vi "MDI-CSM.vi"(7 "Name (\"\" to Use UUID)":string="Event CSM") -> ()   [LabVIEW 2020]
uses:
  Ctl/View.ctl
  <vilib>/Utility/miscctls.llb/LVPoint32TypeDef.ctl
  Ctl/UpdateInsertableVICtl.ctl
  <vilib>/Utility/miscctls.llb/LVPointTypeDef.ctl
  e5d725f2-e4a0-42ba-b3f6-a9ce6c833174.vi
  4b9b3096-98ee-4c27-a851-eb0343d389bf.vi
  ccb737c0-95ef-485f-9e6a-728d6ff02605.vi
  5110686f-90b8-48a6-8112-abce107b1655.vi
  <userlib>/_NEVSTOP/Communicable State Machine(CSM)/AdvanceAPI/CSM - Revert Arguments-Safe String.vi
  <userlib>/_NEVSTOP/Communicable State Machine(CSM)/_Shared/Trim Single-line Text.vi
  <userlib>/_NEVSTOP/Communicable State Machine(CSM)/AdvanceAPI/CSM - Make String Arguments Safe.vi
  <userlib>/_NEVSTOP/Communicable State Machine(CSM)/AdvanceAPI/CSM - Break Down Multiple States String.vi
  <userlib>/_NEVSTOP/Communicable State Machine(CSM)/AdvanceAPI/CSM - Compact Multiple States.vi
  <userlib>/_NEVSTOP/Communicable State Machine(CSM)/AdvanceAPI/CSM - Keywords.vi
  <vilib>/Utility/cursorutil.llb/Set Cursor (Icon Pict).vi
  <userlib>/_NEVSTOP/Communicable State Machine(CSM)/addons/API-String-Arugments-Support/_Support/Convert API String Arguments to Data(variant).vi
  <userlib>/_NEVSTOP/Communicable State Machine(CSM)/Communicable State Machine.lvlib
panel:
  in  "Tab Control 6":T1
  in  "Tab Control 5":T1
  in  "Tab Control 4":T1
  in  "Tab Control 3":T1
  in  "Tab Control 2":T1
  in  "Tab Control":T1
  out "State History":string
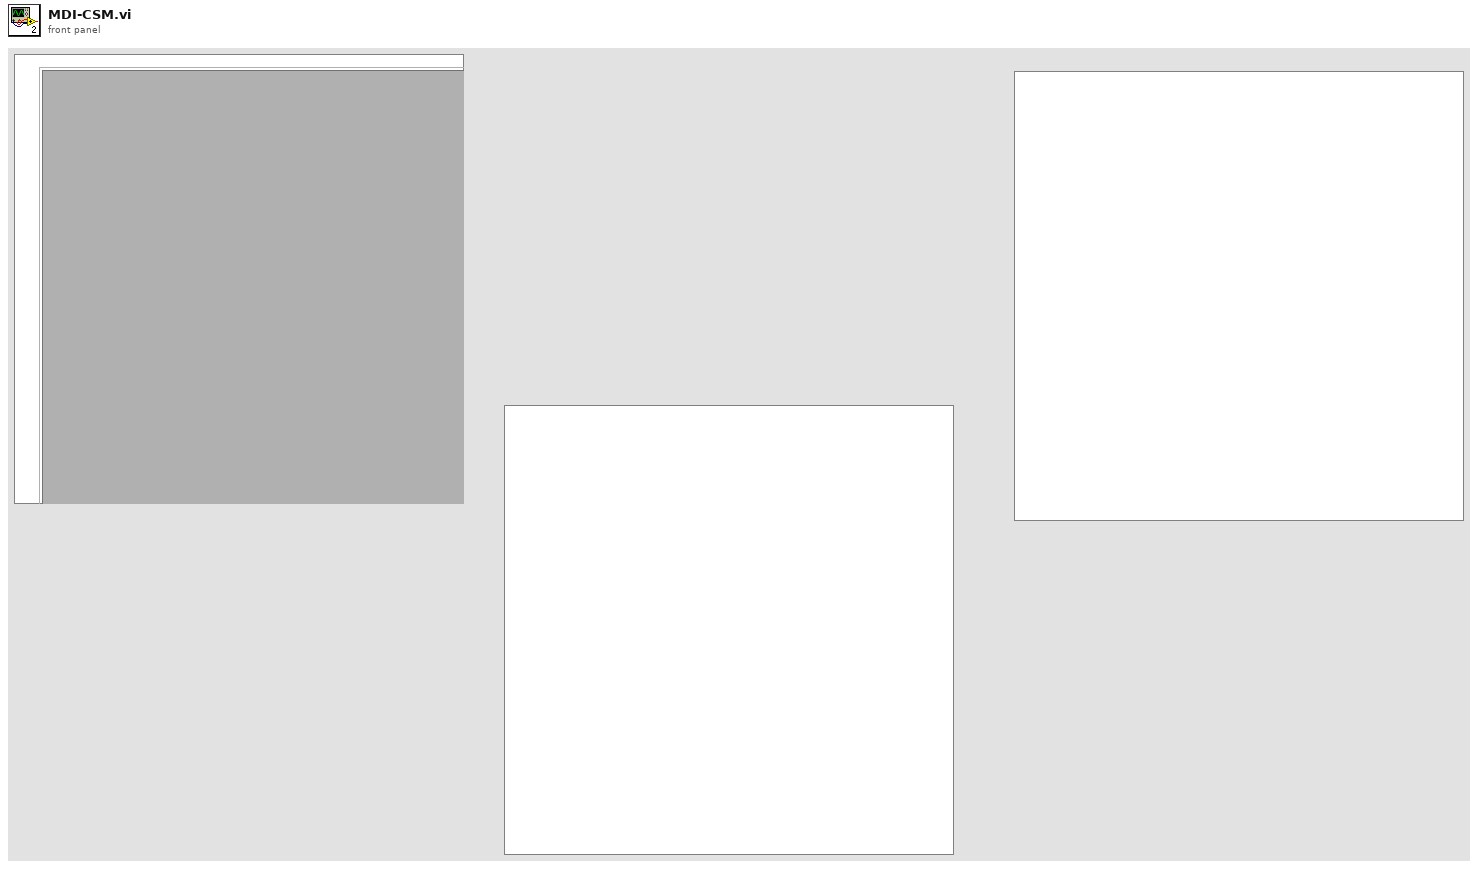
[diagram p1: front panel]
types:
  T1 = typedef "View.ctl" = enum32{"Page 1", "Page 2"}
  T2 = typedef "LVPointTypeDef.ctl" = cluster{"Horizontal":i16, "Vertical":i16}
  T3 = typedef "LVPoint32TypeDef.ctl" = cluster{"Horizontal":i32, "Vertical":i32}
  T4 = typedef "UpdateInsertableVICtl.ctl" = cluster{"Name":string, "VIPath":path}
  T5 = cluster{"Ref":cluster{"TabCtl":refnum<vi>[], "CurrMoveCtl":refnum<vi>, "Pane":refnum<vi>, "SubPanel":refnum<vi>, "Owning VI":refnum<vi>}, "Val":cluster{"TabCtlMove?":bool, "MouseOffset":T3, "UpdateInsertableVI":T4[]}}
  T6 = cluster{"Current VI Reference":refnum<vi>, "Close Panel on Exit?":bool}
  T7 = cluster{"Core":cluster{"Current VI Reference":refnum<vi>, "Close Panel on Exit?":bool}, "1":cluster{"Ref":cluster{"TabCtl":refnum<vi>[], "CurrMoveCtl":refnum<vi>, "Pane":refnum<vi>, "SubPanel":refnum<vi>, "Owning VI":refnum<vi>}, "Val":cluster{"TabCtlMove?":bool, "MouseOffset":T3, "UpdateInsertableVI":T4[]}}}
  T8 = enum32{"Invalid", "Standard", "Closed", "Hidden", "Minimized", "Maximized"}
  T9 = enum32{"invalid app kind", "Development System", "Run Time System", "Student Edition", "Embedded LabVIEW", "Evaluation", "Custom"}
  T10 = typedef "Communicable State Machine.lvlib/_CSM_Response Source Message.ctl" = cluster{"‘State":string, "’Arguments":string, "’Error":errorcluster}
  T11 = typedef "LVPositionTypeDef.ctl" = cluster{"Left":i32, "Top":i32}
  T12 = cluster{"TabCtl":refnum<vi>[], "Pane":refnum<vi>, variant}
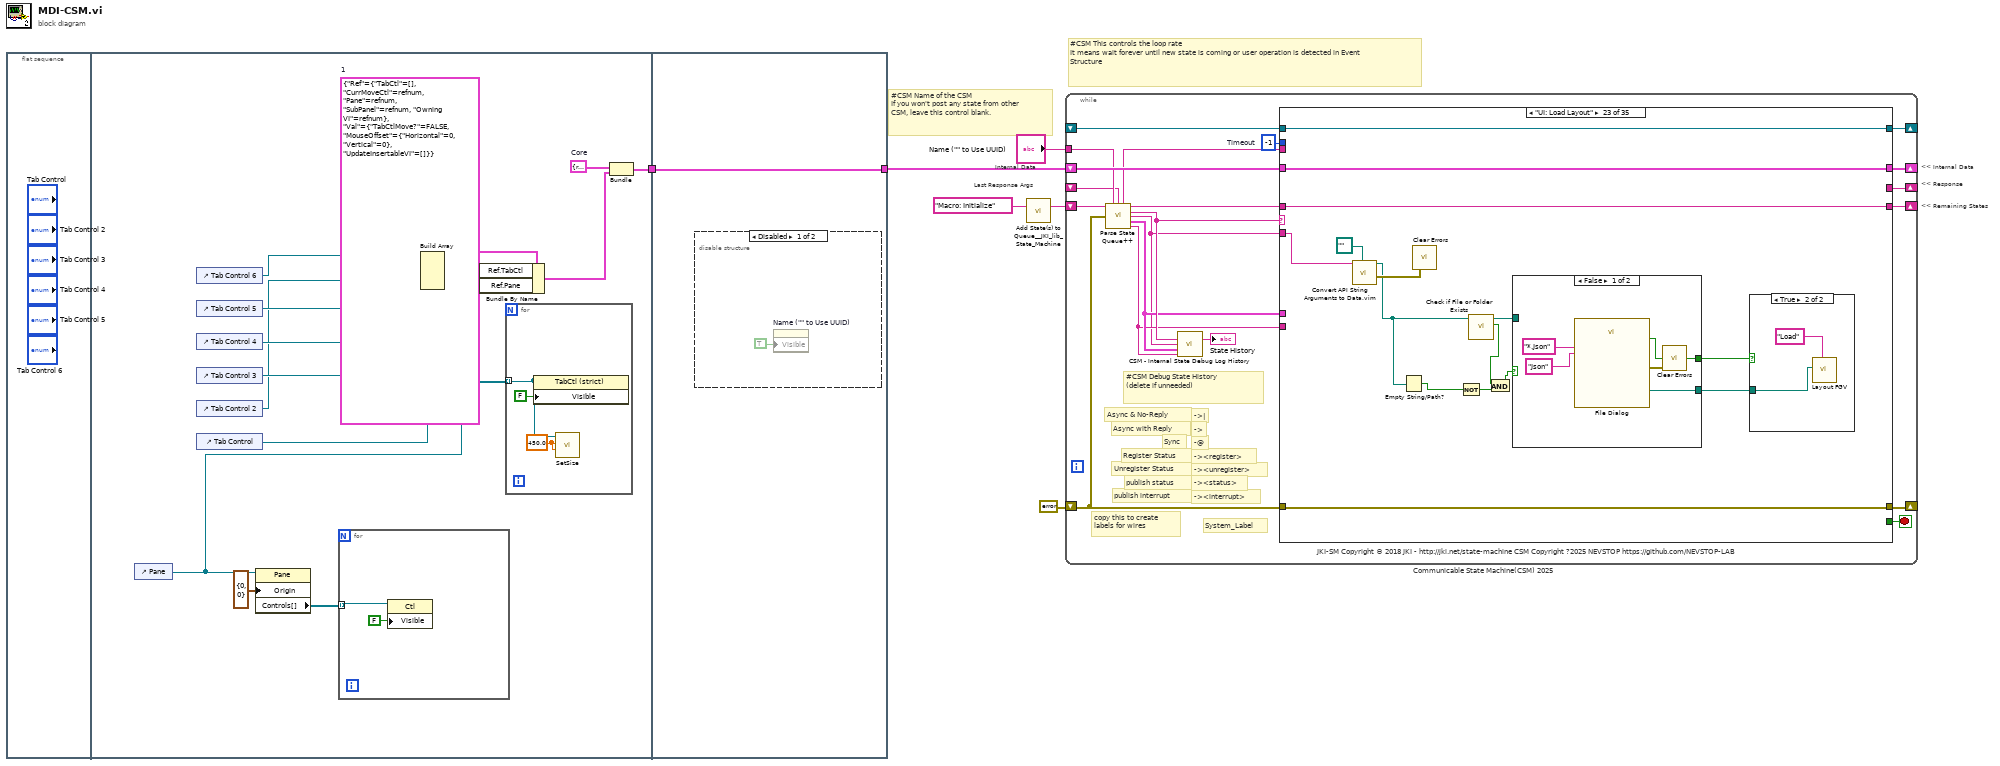
[diagram p0: block diagram]
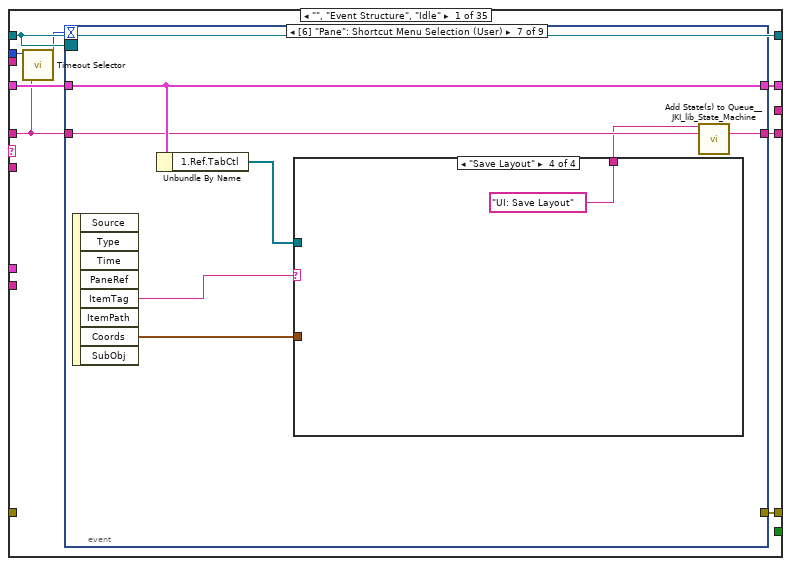
[diagram p2: hidden frame]
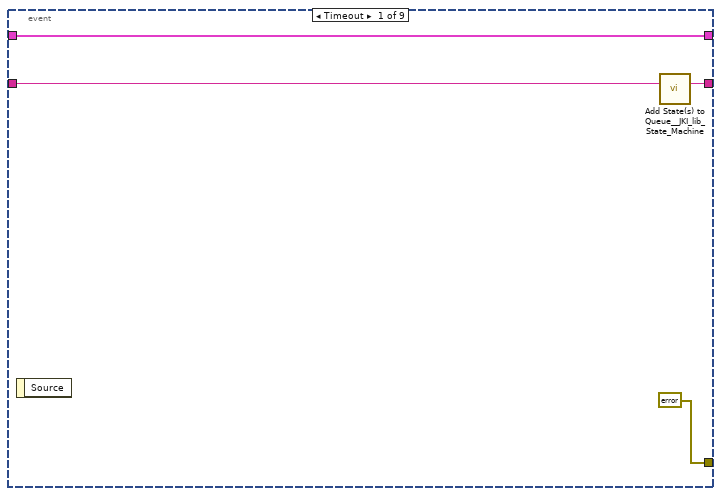
[diagram p3: hidden frame]
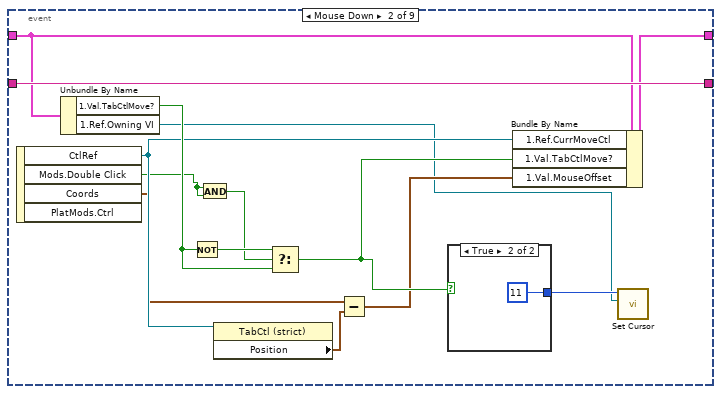
[diagram p4: hidden frame]
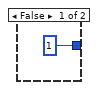
[diagram p5: hidden frame]
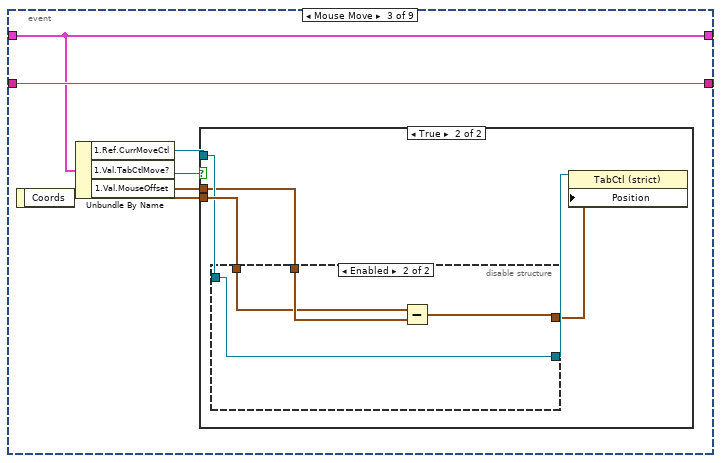
[diagram p6: hidden frame]
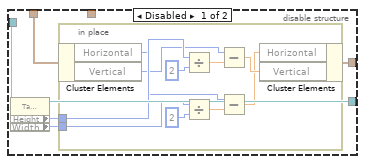
[diagram p8: hidden frame]
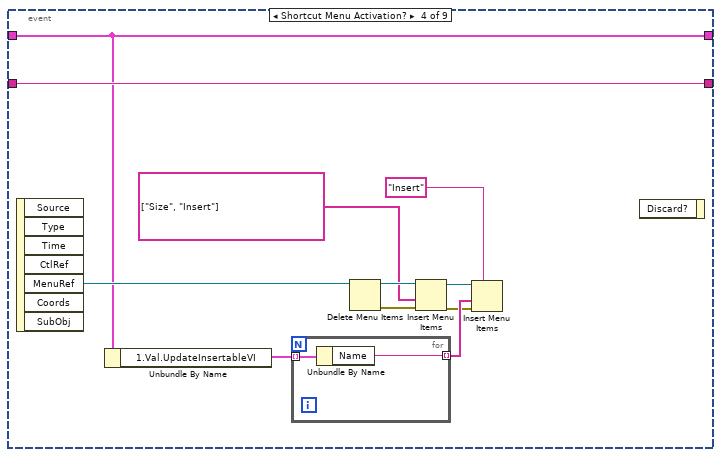
[diagram p9: hidden frame]
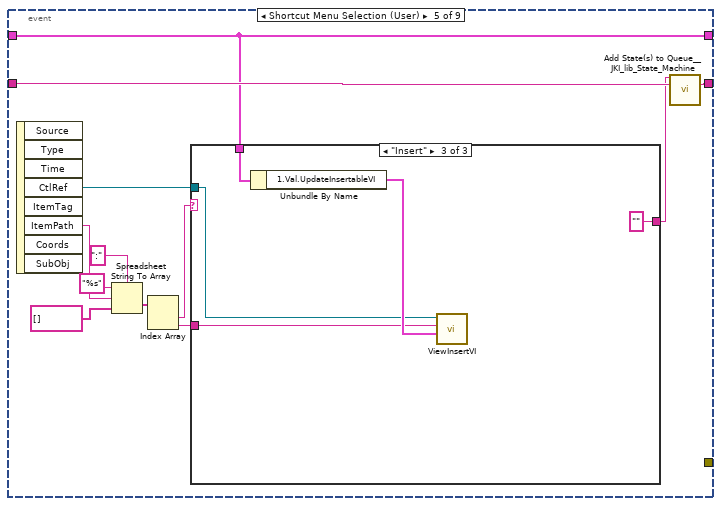
[diagram p10: hidden frame]
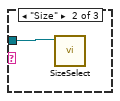
[diagram p12: hidden frame]
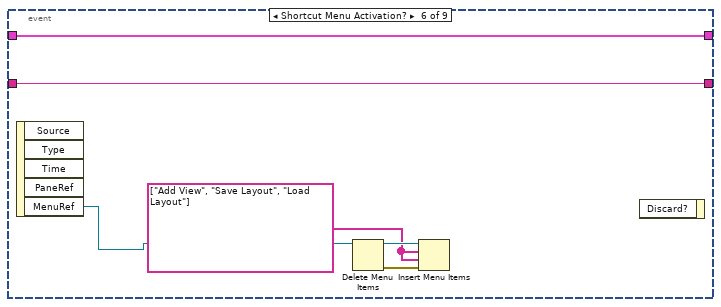
[diagram p13: hidden frame]
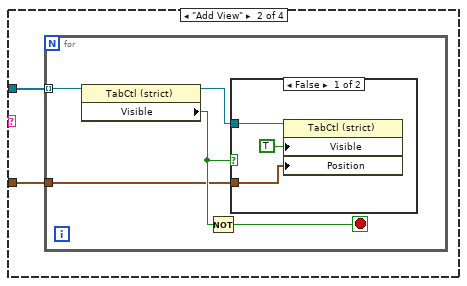
[diagram p15: hidden frame]
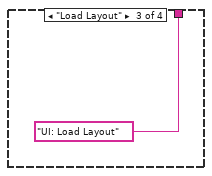
[diagram p17: hidden frame]
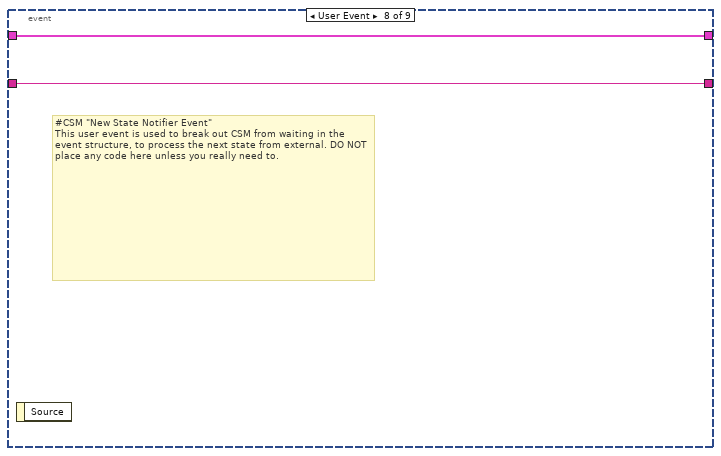
[diagram p18: hidden frame]
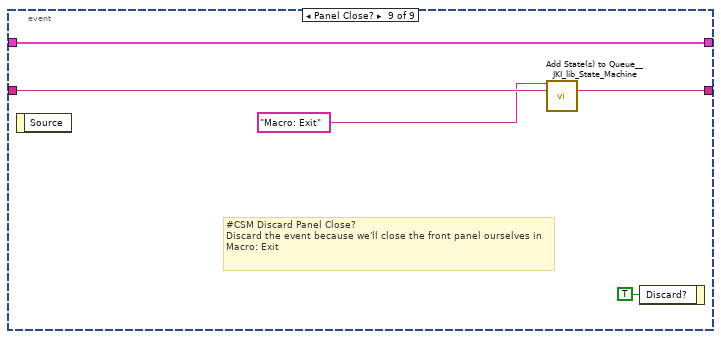
[diagram p19: hidden frame]
diagram:
  # "Last Response Args"
  # "Internal Data"
  # "<< Internal Data"
  # "<< Response"
  # "<< Remaining States"
  # "#CSM Name of the CSM\nIf you won't post any state from other CSM, leave this control blank."
  # "#CSM This controls the loop rate\nIt means wait forever until new state is coming or user operation is detected in Event Structure"
  n1 = flat-sequence {
    tunnel: [w17] -> w1
    tunnel: [w26] -> w2
    tunnel: w1 -> [w26]
    frame #0 {
    }
    frame #1 {
      w19 = T5 {"Ref"={"TabCtl"=[], "CurrMoveCtl"=refnum, "Pane"=refnum, "SubPanel"=refnum, "Owning VI"=refnum}, "Val"={"TabCtlMove?"=FALSE, "MouseOffset"={"Horizontal"=0, "Vertical"=0}, "UpdateInsertableVI"=[]}}  # 1
      w18 = T6 {"Current VI Reference"=refnum, "Close Panel on Exit?"=FALSE}  # Core
      n2 = control-ref of="Pane"() -> (w7:refnum<vi>)
      n3 = control-ref of="Tab Control 6"() -> (w13:refnum<vi>)
      n4 = control-ref of="Tab Control 5"() -> (w12:refnum<vi>)
      n5 = control-ref of="Tab Control 4"() -> (w11:refnum<vi>)
      n6 = control-ref of="Tab Control 3"() -> (w10:refnum<vi>)
      n7 = control-ref of="Tab Control 2"() -> (w9:refnum<vi>)
      n8 = control-ref of="Tab Control"() -> (w8:refnum<vi>)
      n9 = property class="Pane"(reference=w7, "Origin"=T2 {"Horizontal"=0, "Vertical"=0}) -> ("Controls[]"=w14:refnum<vi>[])  [unwired: 1 in, 2 out]
      n10 = for {
        tunnel: w14 -> [w22] mode=indexing
        n11 = property class="Ctl"(reference=w22, "Visible"=FALSE) -> ()  [unwired: 1 in, 2 out]
      }
      n12 = Build Array(w13, w12, w11, w10, w9, w8) -> (w16:refnum<vi>[])
      n13 = Bundle By Name(cluster=w19, "Ref.TabCtl"=w16, "Ref.Pane"=w7) -> (w20:T5)
      n14 = for {
        tunnel: w16 -> [w24] mode=indexing
        w23 = 450.0 ("Height")
        n15 = property class="TabCtl (strict)"(reference=w24, "Visible"=FALSE) -> ()  [unwired: 1 in, 2 out]
        n16 = call "SetSize.vi"("Widht"=w23, "Height"=w23, "TabControl in"=w24) -> ()  [unwired: 9 in]
      }
      n17 = Bundle("Core"=w18, "1"=w20) -> (w17:T7)  [unwired: 1 in]
    }
    frame #2 {
      n18 = disable-structure shown="Disabled" {
        frame Disabled {
          n19 = property on="Name (\"\" to Use UUID)" class="Str"("Visible"=TRUE) -> ()  [unwired: 2 in, 2 out]
        }
        frame Enabled {
        }
      }
    }
  }
  n20 = call <vilib>:"Add State(s) to Queue__JKI_lib_State_Machine.vi"("State(s) in (\"\")"="Macro: Initialize" ("Init State(\"Macro: Initialize\")")) -> ("States Out"=w3:string)  [unwired: 14 in]
  n21 = while "Communicable State Machine(CSM) 2025" {
    shift-right: [w42] -> _
    shift-left: w2 -> [w41]
    shift-right: [w45] -> _
    shift-left: errorcluster {"status"=FALSE, "code"=0, "source"=""} ("error out") -> [w39]
    shift-right: [w44] -> _
    shift-left: w3 -> [w46]
    tunnel: "Name (\"\" to Use UUID)" -> [w35]
    shift-right: [w38] -> _
    shift-left: _ -> [w30]
    shift-right: [w37] -> _
    shift-left: _ -> [w36]
    stop <- w43 stop-if-true
    w40 = -1  # Timeout
    # "#CSM Debug State History\n(delete if unneeded)"
    # "-><interrupt>"
    # "-><status>"
    # "-><unregister>"
    # "-><register>"
    # "-@"
    # "->"
    # "->|"
    # "publish interrupt"
    # "publish status"
    # "Unregister Status"
    # "Register Status"
    # "Sync"
    # "Async with Reply"
    # "Async & No-Reply"
    # "copy this to create labels for wires"
    # "System_Label"
    # "JKI-SM Copyright © 2018 JKI - http://jki.net/state-machine CSM Copyright ?2025 NEVSTOP https://github.com/NEVSTOP-LAB"
    n22 = call <userlib>:"Parse State Queue++.vi"("State Queue"=w46, "Name (\"\" to Use UUID)"=w35, "Response Arguments"=w30, "Previous Error"=w39) -> ("Name Used"=w31:string, "Remaining States"=w47:string, "Current State"=w34:string, "Arguments"=w29:string, "Additional Information"=w33:T10, "Source CSM"=w32:string)  [unwired: 6 in]
    n23 = call <userlib>:"CSM - Internal State Debug Log History.vi"("State"=w34, "Arguments (\"\")"=w29, ">> Response Source Message >>"=w33, "Source (\"\")"=w32) -> ("Debug Log"=→"State History":string)  [unwired: 11 in]
    n24 = case shown="\"UI: Load Layout\"" w34 {
      selector: w34 -> [_ _ _ w180 _ _ _ _ _ _ _ _ _ _ _ _ _ _ _ _ _ _ _ _ _ _ _ _ _ _ _ _ _ _ _]
      tunnel: w47 -> [w48 w172 w177 w186 w192 w198 w224 w232 w239 w249 w258 w271 w276 w280 w284 w290 w294 w304 w308 w312 w321 w335 w359 w375 w386 w450 w455 w466 w469 w478 w483 w495 w499 w503 w507]
      tunnel: w29 -> [_ _ _ _ _ w196 w220 w227 w235 w243 _ _ _ _ _ _ _ _ _ _ _ w332 w355 w371 w381 _ _ _ _ w475 w480 w493 _ _ _]
      tunnel: w41 -> [w54 w171 w174 w184 w191 w204 w225 w230 w237 w247 w257 w265 w274 w278 w281 w286 w292 w296 w307 w310 w314 w333 w357 w373 w383 w448 w453 w464 w468 w477 w482 w489 w497 w501 w505]
      tunnel: [w53 _ w175 w178 w193 errorcluster {"status"=FALSE, "code"=0, "source"=""} ("error out") w217 w226 w233 w246 _ _ _ _ _ w287 _ w299 w306 _ _ w336 w360 w372 w384 _ _ _ _ _ _ _ _ _ _] -> w45
      tunnel: w39 -> [_ _ w175 w179 w193 w202 w218 w228 w234 _ _ _ _ _ _ _ _ _ _ _ _ w336 w360 _ _ _ _ _ _ _ _ _ _ _ _]
      tunnel: [w55 w172 w176 w185 w192 w200 w223 w231 w238 w250 w258 w270 w275 w279 w283 w289 w293 w304 w308 w311 w320 w335 w359 w374 w385 w449 w454 w465 w469 w478 w483 w495 w498 w502 w506] -> w44
      tunnel: [_ _ _ _ _ _ TRUE _ _ _ _ _ TRUE _ _ _ _ _ _ _ _ _ _ _ _ _ _ _ _ _ _ _ _ _ _] -> w43
      tunnel: [w52 w171 w174 w184 w191 w204 w225 w230 w237 w248 w257 w269 w274 w278 w281 w286 w292 w296 w307 w310 w314 w333 w357 w373 w383 w448 w453 w464 w468 w473 w482 w487 w497 w501 w505] -> w42
      tunnel: w40 -> [w50 _ _ _ _ _ _ _ _ _ _ _ _ _ _ _ _ _ _ _ _ _ _ _ _ _ _ _ _ _ _ _ _ _ _]
      tunnel: w32 -> [_ _ _ _ _ w195 _ _ _ w244 _ _ _ _ _ _ _ _ _ _ _ _ _ _ _ _ _ _ _ _ _ _ _ _ _]
      tunnel: w33 -> [_ _ _ _ _ w194 _ _ _ w245 _ _ _ _ _ _ _ _ _ _ _ _ _ _ _ _ _ _ _ _ _ _ _ _ _]
      tunnel: [_ _ _ "" w187 _ _ _ _ _ _ _ _ _ _ _ _ _ _ _ _ _ _ _ _ _ _ _ _ _ _ _ _ _ _] -> w38
      tunnel: [w51 w170 w173 w182 w190 w203 w221 w229 w236 w251 w256 w259 w272 w277 w282 w285 w291 w303 w305 w309 w319 w334 w358 w370 w380 w447 w451 w457 w467 w476 w481 w494 w496 w500 w504] -> w37
      tunnel: w36 -> [w51 w170 w173 w182 w190 w203 w221 w229 w236 w251 w256 w259 w272 w277 w282 w285 w291 _ w305 w309 w319 w334 w358 w370 w380 w447 w451 w457 w467 w476 w481 w494 w496 w500 w504]
      tunnel: w31 -> [_ _ _ w181 _ _ w219 _ _ _ _ _ _ _ _ _ _ w302 _ _ _ _ _ _ _ _ _ _ _ _ _ _ _ _ _]
      frame "", "Event Structure", "Idle" {
        n25 = call <userlib>:"Timeout Selector.vi"("Remaining States"=w48, "Timeout Expected"=w50) -> ("Timeout"=w49:i32)  [unwired: 5 in]
        n26 = event shown="[6] \"Pane\": Shortcut Menu Selection (User)" {
          selector: w51 -> [_ _ _ _ _ _ _ _ _]
          dyn-events: _ -> [_ _ _ _ _ _ _ _ _]
          timeout: w49 -> [_ _ _ _ _ _ _ _ _]
          tunnel: w48 -> [w59 w73 w81 w117 w130 w143 w147 w163 w169]
          tunnel: [w58 w73 w81 w117 w129 w143 w146 w163 w168] -> w55
          tunnel: w54 -> [w57 w70 w79 w111 w120 w142 w149 w164 w167]
          tunnel: [errorcluster {"status"=FALSE, "code"=0, "source"=""} ("error out") _ _ _ _ _ _ _ _] -> w53
          tunnel: [w57 w68 w79 w111 w120 w142 w149 w164 w167] -> w52
          event Timeout {
            n27 = event-data() -> ()  [unwired: 1 in, 1 out]
            n28 = call <vilib>:"Add State(s) to Queue__JKI_lib_State_Machine.vi"("State(s) in (\"\")"=w59) -> ("States Out"=w58:string)  [unwired: 14 in]
          }
          event Mouse Down {
            n29 = event-data() -> ("CtlRef"=w66:refnum<vi>, "Mods.Double Click"=w60:bool, "Coords"=w64:T3)  [unwired: 1 in, 1 out]
            n30 = Unbundle By Name(w70) -> ("1.Val.TabCtlMove?"=w69:bool, "1.Ref.Owning VI"=w62:refnum<vi>)
            n31 = Not(x=w69) -> (.not. x?=w72:bool)
            n32 = And(x=w60, y=w60) -> (x .and. y?=w61:bool)
            n33 = property class="TabCtl (strict)"(reference=w66) -> ("Position"=w65:T11)  [unwired: 1 in, 2 out]
            n34 = Select(t=w72, s=w61, f=w69) -> (s? t:f=w67:bool)
            n35 = Subtract(x=w64, y=w65) -> (x-y=w63:T3)
            n36 = case shown="True" w67 {
              tunnel: [u16 1 ("icon") u16 11 ("icon")] -> w71
              frame False {
              }
              frame True {
              }
            }
            n37 = Bundle By Name(cluster=w70, "1.Ref.CurrMoveCtl"=w66, "1.Val.TabCtlMove?"=w67, "1.Val.MouseOffset"=w63) -> (w68:T7)
            n38 = call-poly <vilib>:"Set Cursor.vi"("VI reference (current VI)"=w62, "icon"=w71) -> ()  [unwired: 8 in, 2 out]
          }
          event Mouse Move {
            n39 = event-data() -> ("Coords"=w80:T3)  [unwired: 1 in]
            n40 = Unbundle By Name(w79) -> ("1.Ref.CurrMoveCtl"=w77:refnum<vi>, "1.Val.TabCtlMove?"=w78:bool, "1.Val.MouseOffset"=w76:T3)
            n41 = case shown="True" w78 {
              tunnel: w80 -> [_ w86]
              tunnel: w77 -> [_ w85]
              tunnel: w76 -> [_ w82]
              frame False {
              }
              frame True {
                n42 = disable-structure shown="Enabled" {
                  disable-tunnel: w86 -> [w90 w104]
                  disable-tunnel: w85 -> [w89 w106]
                  disable-tunnel: [w88 w106] -> w84
                  disable-tunnel: [w87 w103] -> w83
                  disable-tunnel: w82 -> [_ w105]
                  frame Disabled {
                    n43 = property class="TabCtl (strict)"(reference=w89) -> (reference out=w88:refnum<vi>, "Height"=w92:u32, "Width"=w91:u32)  [unwired: 1 in, 1 out]
                    n44 = in-place {
                      in-place-border: w92 -> [w102]
                      in-place-border: w91 -> [w96]
                      n45 = in-place-cluster #1(w90) -> ("Horizontal"=w94:i32, "Vertical"=w93:i32)
                      n46 = Divide(x=w102, y=u32 2) -> (x/y=w100:dbl)
                      n47 = Divide(x=w96, y=u32 2) -> (x/y=w97:dbl)
                      n48 = Subtract(x=w93, y=w100) -> (x-y=w99:dbl)
                      n49 = Subtract(x=w94, y=w97) -> (x-y=w95:dbl)
                      n50 = in-place-cluster #1("Horizontal"=w95, "Vertical"=w99) -> (w87:T3)
                    }
                  }
                  frame Enabled {
                    n51 = Subtract(x=w104, y=w105) -> (x-y=w103:T3)
                  }
                }
                n52 = property class="TabCtl (strict)"(reference=w84, "Position"=w83) -> ()  [unwired: 1 in, 2 out]
              }
            }
          }
          event Shortcut Menu Activation? {
            n53 = event-data() -> ("MenuRef"=w113:refnum<k9>)  [unwired: 1 in, 6 out]
            n54 = Unbundle By Name(w111) -> ("1.Val.UpdateInsertableVI"=w110:T4[])
            n55 = for {
              tunnel: w110 -> [w119] mode=indexing
              tunnel: [w118] -> w109 mode=indexing
              n56 = Unbundle By Name(w119) -> ("Name"=w118:string)
            }
            n57 = Delete Menu Items(9:w113) -> (0:w116:errorcluster, 3:w115:refnum<k9>)  [unwired: 3 in]
            n58 = Insert Menu Items(6:w116, 7:string[] ["Size", "Insert"] ("item names"), 9:w115) -> (0:w107:errorcluster, 3:w108:refnum<k9>)  [unwired: 3 in, 1 out]
            n59 = Insert Menu Items(5:"Insert", 6:w107, 7:w109, 9:w108) -> ()  [unwired: 2 in, 3 out]
            n60 = event-data() -> ()  [unwired: 2 in, 1 out]
          }
          event Shortcut Menu Selection (User) {
            n61 = event-data() -> ("CtlRef"=w131:refnum<vi>, "ItemPath"=w126:string)  [unwired: 1 in, 6 out]
            n62 = Spreadsheet String To Array(delimiter (Tab)=":", format string="%s", spreadsheet string=w126, array type (2D Dbl)=string[] [] ("delimiter (Tab)")) -> (array=w123:string[])
            n63 = Index Array(array=w123) -> (element #1=w122:string, element #2=w121:string)  [unwired: 2 in]
            n64 = case shown="\"Insert\"" w122 {
              tunnel: w131 -> [_ w132 w134]
              tunnel: [_ _ "" ("State(s) in Front (\"\")")] -> w128
              tunnel: w121 -> [_ _ w135]
              tunnel: w120 -> [_ _ w137]
              frame "False", Default {
              }
              frame "Size" {
                n65 = call "SizeSelect.vi"("CtlRef"=w132) -> ()  [unwired: 11 in]
              }
              frame "Insert" {
                n66 = Unbundle By Name(w137) -> ("1.Val.UpdateInsertableVI"=w136:T4[])
                n67 = call "ViewInsertVI.vi"("UpdateInsertableVI"=w136, "Name"=w135, "TabControl in"=w134) -> ()  [unwired: 9 in]
              }
            }
            n68 = call <vilib>:"Add State(s) to Queue__JKI_lib_State_Machine.vi"("State(s) in Front (\"\")"=w128, "State(s) in (\"\")"=w130) -> ("States Out"=w129:string)  [unwired: 13 in]
          }
          event Shortcut Menu Activation? {
            w139 = string[] ["Add View", "Save Layout", "Load Layout"] ("item names")
            n69 = event-data() -> ("MenuRef"=w138:refnum<k9>)  [unwired: 1 in, 4 out]
            n70 = Delete Menu Items(9:w138) -> (0:w141:errorcluster, 3:w140:refnum<k9>)  [unwired: 3 in]
            n71 = Insert Menu Items(6:w141, 7:w139, 8:w139, 9:w140) -> ()  [unwired: 2 in, 3 out]
            n72 = event-data() -> ()  [unwired: 2 in, 1 out]
          }
          event Shortcut Menu Selection (User) {
            n73 = event-data() -> ("ItemTag"=w150:string, "Coords"=w144:T3)  [unwired: 1 in, 6 out]
            n74 = Unbundle By Name(w149) -> ("1.Ref.TabCtl"=w148:refnum<vi>[])
            n75 = case shown="\"Save Layout\"" w150 {
              tunnel: w148 -> [_ w152 _ _]
              tunnel: w144 -> [_ w151 _ _]
              tunnel: [_ _ "UI: Load Layout" ("State(s) in Front (\"\")") "UI: Save Layout" ("State(s) in Front (\"\")")] -> w145
              frame "False", Default {
              }
              frame "Add View" {
                n76 = for {
                  tunnel: w152 -> [w157] mode=indexing
                  tunnel: w151 -> [w153]
                  stop <- w155 stop-if-true
                  n77 = property class="TabCtl (strict)"(reference=w157) -> (reference out=w154:refnum<vi>, "Visible"=w156:bool)  [unwired: 1 in, 1 out]
                  n78 = Not(x=w156) -> (.not. x?=w155:bool)
                  n79 = case shown="False" w156 {
                    tunnel: w154 -> [w160 _]
                    tunnel: w153 -> [w158 _]
                    frame False {
                      n80 = property class="TabCtl (strict)"(reference=w160, "Visible"=TRUE, "Position"=w158) -> ()  [unwired: 1 in, 2 out]
                    }
                    frame True {
                    }
                  }
                }
              }
              frame "Load Layout" {
              }
              frame "Save Layout" {
              }
            }
            n81 = call <vilib>:"Add State(s) to Queue__JKI_lib_State_Machine.vi"("State(s) in Front (\"\")"=w145, "State(s) in (\"\")"=w147) -> ("States Out"=w146:string)  [unwired: 13 in]
          }
          event User Event {
            # "#CSM \"New State Notifier Event\"\nThis user event is used to break out CSM from waiting in the event structure, to process the next state from external. DO NOT place any code here unless you really need to."
            n82 = event-data() -> ()  [unwired: 1 in, 1 out]
          }
          event Panel Close? {
            # "#CSM Discard Panel Close?\nDiscard the event because we'll close the front panel ourselves in Macro: Exit"
            n83 = event-data() -> ()  [unwired: 1 in, 1 out]
            n84 = call <vilib>:"Add State(s) to Queue__JKI_lib_State_Machine.vi"("State(s) in Front (\"\")"="Macro: Exit", "State(s) in (\"\")"=w169) -> ("States Out"=w168:string)  [unwired: 13 in]
            n85 = event-data("Discard?"=TRUE) -> ()  [unwired: 1 in, 1 out]
          }
        }
      }
      frame "CSM Documentation" {
        # "#CSM State Syntax\n\n// Comment line, all text to the right of “//” will be ignored\n// Local Message Example\nDoSth: DoA >> Arguments\n\n// Sync Call Example\nAPI: xxxx >> Arguments -@ TargetModule\n\n// Async Call Example\nAPI: xxxx >> Arguments -> TargetModule\n\n// Async Call without Reply Example\nAPI: xxxx >> Arguments ->| TargetModule\n\n// Broadcast normal status:\nStatus >> StatusArguments  -><status>\n\n// Broadcast Interrupt status:\nInterrupt >> StatusArguments  -><interrupt>\n\n// Register Source Module's status to Handler Module\nStatus@Source Module >> Handler Module@Handler Module -><register>\n\n// Unegister Source Module's status\nStatus@Source Module >> Handler Module -><unregister>"
        # "#CSM README FIRST\n\nCommunicable State Machine(CSM) is a LabVIEW application framework that builds upon JKI State Machine(JKISM). It follows the pattern of JKISM and extends the keywords to describe message communication between modules, including concepts such as Sync-Message, Async-Message, Subscription/Unsubscription of status - essential elements for creating reusable code modules. For more information, please visit the CSM wiki: https://nevstop-lab.github.io/CSM-Wiki/\n\nFor instructions on JKI State Machine, visit: \n    http://jki.net/state-machine/\nFor information about CSM, visit: \n    https://github.com/NEVSTOP-LAB"
        # "#CSM \"Documentation\"\nCase for holding CSM Documenation"
      }
      frame "---------- Core ----------" {
        # "#CSM \"Category Seperator\"\nDo not put any code in this frame."
        n86 = call <vilib>:"Add State(s) to Queue__JKI_lib_State_Machine.vi"("State(s) in (\"\")"=w177) -> ("States Out"=w176:string)  [unwired: 14 in]
      }
      frame Default {
        # "#CSM \"Default\"\nthis is used to capture unhandled states and typos"
        n87 = call <userlib>:"CSM Unhandled State Error.vi"("error in (no error)"=w179, "Undefined State"=w180, "CSM Name"=w181) -> ("error out"=w178:errorcluster)  [unwired: 8 in]
        n88 = call <vilib>:"Add State(s) to Queue__JKI_lib_State_Machine.vi"("State(s) in (\"\")"=w186) -> ("States Out"=w185:string)  [unwired: 14 in]
      }
      frame "VI Reference" {
        n89 = Unbundle By Name(w191) -> ("Core"=w189:T6)
        n90 = Unbundle By Name(w189) -> ("Current VI Reference"=w188:refnum<vi>)
        n91 = call <userlib>:"CSM - Convert Data to HexStr.vi"("Variant"=w188) -> ("HEX String (0-9,A-F)"=w187:string)  [unwired: 8 in]
      }
      frame "Error Handler" {
        # "#CSM Disable this error dialog if you need"
        # "#CSM \"Error Handler\"\nYou can also output any states to clean-up after errors occur"
        # "Clear error"
        n92 = case shown="Error" w202 {
          selector: w202 -> [_ w211]
          tunnel: [w209 w213] -> w199
          tunnel: w198 -> [w209 w212]
          tunnel: [w208 w211] -> w197
          tunnel: w196 -> [w210 _]
          tunnel: w195 -> [_ _]
          tunnel: w194 -> [_ _]
          frame No Error {
            n93 = call <userlib>:"CSM - Convert Argument to Error.vi"("Argument"=w210) -> ("Error"=w208:errorcluster)  [unwired: 4 in]
            n94 = flat-sequence {
              frame #0 {
                # "#CSM External Error Handler Case\nUsually, it's because This CSM register others' \"Error Occurred\" status with \"Error Handler\". If other CSM have any error, the error will be passed here for central handling."
              }
            }
          }
          frame Error {
            # "#CSM Internal Error Handler Case \nIf any error Occurred, \"Error Occurred\" \nstatus update will be broadcasted to system.\nParameter is Error Cluster."
            n95 = call <userlib>:"CSM - Convert Error to Argument.vi"("Error"=w211) -> ("Argument"=w215:string)  [unwired: 4 in]
            n96 = call <vilib>:"Build State String with Arguments__JKI_lib_State_Machine.vi"("Arguments (\"\")"=w215, "State"="Error Occurred" ("Status with Arguments")) -> ("State with Arguments"=w214:string)  [unwired: 4 in]
            n97 = call <userlib>:"CSM - Broadcast Status Change.vi"("Status With Arguments"=w214, "State Queue"=w212) -> ("Remaining States"=w213:string)  [unwired: 13 in]
          }
        }
        n98 = disable-structure shown="Enabled" {
          disable-tunnel: w197 -> [w206 w207]
          frame Enabled {
            # "Unhandled Error -- Display it"
            n99 = call <vilib>:"General Error Handler.vi"("error in (no error)"=w206) -> ()  [unwired: 10 in, 5 out]
          }
          frame Disabled {
            n100 = call <vilib>:"Clear Errors.vi"("error in (no error)"=w207) -> ()  [unwired: 5 in, 2 out]
          }
        }
        n101 = call <vilib>:"Add State(s) to Queue__JKI_lib_State_Machine.vi"("State(s) in Front (\"\")"="// Post Error States", "State(s) in (\"\")"=w199) -> ("States Out"=w200:string)  [unwired: 13 in]
      }
      frame "Critical Error" {
        # "#CSM \"Critical Error\"\nWhen any un-recoverable error occurs, CSM goes into this case."
        # "#CSM Stop in Critical Error\nWhen Critical Error occurs, Stop the loop immediately. Do NOT change this unless you fully understand the impact."
        n102 = call <userlib>:"CSM Critical Error.vi"("error in (no error)"=w218, "Arugments (As Reason)"=w220, "CSM Name"=w219) -> ("error out"=w217:errorcluster)  [unwired: 8 in]
        n103 = call <vilib>:"Add State(s) to Queue__JKI_lib_State_Machine.vi"("State(s) in (\"\")"=w224) -> ("States Out"=w223:string)  [unwired: 14 in]
      }
      frame "Target Timeout Error" {
        # "#CSM \"Target Timeout Error\"\nWhen This CSM could not get the sync-call response in time, This CSM goes into this case."
        n104 = call <userlib>:"CSM Target Timeout Error.vi"("error in (no error)"=w228, "Arguments (As CSM Name)"=w227) -> ("error out"=w226:errorcluster)  [unwired: 9 in]
        n105 = call <vilib>:"Add State(s) to Queue__JKI_lib_State_Machine.vi"("State(s) in (\"\")"=w232) -> ("States Out"=w231:string)  [unwired: 14 in]
      }
      frame "Target Error" {
        # "#CSM \"Target Error\"\nWhen This CSM try to communicate with an un-existed CSM, This CSM goes into this case."
        n106 = call <userlib>:"CSM Target Error.vi"("error in (no error)"=w234, "Arguments (As CSM Name)"=w235) -> ("error out"=w233:errorcluster)  [unwired: 9 in]
        n107 = call <vilib>:"Add State(s) to Queue__JKI_lib_State_Machine.vi"("State(s) in (\"\")"=w239) -> ("States Out"=w238:string)  [unwired: 14 in]
      }
      frame "Async Response", "Response" {
        # "#CSM \"Async Response\"\nHandle Async-call Response (\"Async Response\" for ->)"
        # "#CSM \"Response\"\nHandle Sync-call Response (\"Response\" for -@)"
        n108 = Unbundle(w245) -> ("‘State"=w242:string, "’Arguments"=w241:string, "’Error"=w240:errorcluster)
        n109 = case shown="Default" w242 {
          tunnel: [w252] -> w250
          tunnel: w249 -> [w253]
          tunnel: [w255] -> w248
          tunnel: w247 -> [w255]
          tunnel: [w254] -> w246
          tunnel: w240 -> [w254]
          tunnel: w244 -> [_]
          tunnel: w243 -> [_]
          tunnel: w241 -> [_]
          frame Default {
            # "#CSM Response Comments\nAfter Message is executed, CSM goes to this state for receive the response.\n    For Async Message(->), \"Async Response\" is used. This CSM will goes to \"Async Message Posted\" immediately and receive the \"Async Response\" after the callee finishes the message.\n    For Sync Message(@),  This CSM will wait until the message is done and immediately goes to \"Response\""
            n110 = call <vilib>:"Add State(s) to Queue__JKI_lib_State_Machine.vi"("State(s) in (\"\")"=w253) -> ("States Out"=w252:string)  [unwired: 14 in]
          }
        }
      }
      frame "Async Message Posted" {
        # "#CSM \"Async Message Posted\"\nAfter Async Message is posted (-> or ->| ), CSM goes to this state for post-action.\nYou can use Argument - State to tell which Async Message is called."
      }
      frame "Initialize Core Data" {
        # "#CSM \"Initialize Core Data\"\nThis is used to determine panel behavior on exit"
        # "originally closed?"
        # "exe?"
        # "If panel starts closed or is an EXE, then close it when we exit"
        n111 = property class="VI"() -> ("FP.State"=w262:T8)  [unwired: 2 in, 2 out]
        n112 = property class="App"() -> ("App.Kind"=w268:T9)  [unwired: 2 in, 2 out]
        n113 = control-ref of="Current VI Reference"() -> (w263:refnum<vi>)
        n114 = Equal?(x=w262, y=T8."Closed" ("Front Panel Window:State")) -> (x = y?=w260:bool)
        n115 = Equal?(x=w268, y=T9."Run Time System" ("Application:Kind")) -> (x = y?=w266:bool)
        n116 = Or(x=w260, y=w266) -> (x .or. y?=w264:bool)
        n117 = Bundle By Name(cluster=w265, "Core.Current VI Reference"=w263, "Core.Close Panel on Exit?"=w264) -> (w269:T7)
        n118 = call <vilib>:"Add State(s) to Queue__JKI_lib_State_Machine.vi"("State(s) in (\"\")"=w271) -> ("States Out"=w270:string)  [unwired: 14 in]
      }
      frame "Exit" {
        # "#CSM \"Exit\"\nCase for exiting the loop. No errors that occur here will be handled."
        n119 = call <vilib>:"Add State(s) to Queue__JKI_lib_State_Machine.vi"("State(s) in (\"\")"=w276) -> ("States Out"=w275:string)  [unwired: 14 in]
      }
      frame "---------- Data ----------" {
        # "#CSM \"Category Seperator\"\nDo not put any code in this frame."
        n120 = call <vilib>:"Add State(s) to Queue__JKI_lib_State_Machine.vi"("State(s) in (\"\")"=w280) -> ("States Out"=w279:string)  [unwired: 14 in]
      }
      frame "Data: Initialize" {
        # "#CSM \"Data: Initialize\"\nInitialize the shift-register data, here.\n(data names are defined by what you wire into the bundle function)"
        n121 = call <vilib>:"Add State(s) to Queue__JKI_lib_State_Machine.vi"("State(s) in (\"\")"=w284) -> ("States Out"=w283:string)  [unwired: 14 in]
      }
      frame "Data: Cleanup" {
        # "#CSM \"Data: Cleanup\"\nCleanup any data and references, here.\n(this is called automatically, by the Macro: Exit)"
        n122 = Unbundle By Name(w286) -> ("Core.Current VI Reference"=w288:refnum<vi>)
        n123 = Close Reference(reference=w288) -> (error out=w287:errorcluster)  [unwired: 1 in]
        n124 = call <vilib>:"Add State(s) to Queue__JKI_lib_State_Machine.vi"("State(s) in (\"\")"=w290) -> ("States Out"=w289:string)  [unwired: 14 in]
      }
      frame "---------- Events ----------" {
        # "#CSM \"Category Seperator\"\nDo not put any code in this frame."
        n125 = call <vilib>:"Add State(s) to Queue__JKI_lib_State_Machine.vi"("State(s) in (\"\")"=w294) -> ("States Out"=w293:string)  [unwired: 14 in]
      }
      frame "Events: Register" {
        w298 = cluster{"TabCtl":refnum<vi>[]} {"TabCtl"=[]}  # TabCtlEvent
        # "#CSM \"Events: Register\"\nRegister user event. New Message Event is registered to break CSM waiting in event structure by default."
        # "#CSM Register New Message Event\nRegister message event to break Waiting in Event structure."
        n126 = Unbundle By Name(w296) -> ("1.Ref.TabCtl"=w295:refnum<vi>[])
        n127 = Bundle By Name(cluster=w298, "TabCtl"=w295) -> (w297:cluster{"TabCtl":refnum<vi>[]})
        n128 = call <userlib>:"CSM - Get New State Notifier Event.vi"("Name (\"\" to Use UUID)"=w302) -> ("error out"=w300:errorcluster, "New State Notifier Event"=w301:refnum<user-event>)  [unwired: 9 in]
        n129 = register-events(error in=w300, w301, w297, w297, w297) -> (reference out=w303:refnum<event-registration>, error out=w299:errorcluster)  [unwired: 1 in]
      }
      frame "Events: Unregister" {
        # "#CSM \"Events: Unregister\"\nUnregister user event."
        n130 = Unregister For Events(event registration refnum=w305) -> (error out=w306:errorcluster)  [unwired: 1 in]
      }
      frame "---------- UI ----------" {
        # "#CSM \"Category Seperator\"\nDo not put any code in this frame."
        n131 = call <vilib>:"Add State(s) to Queue__JKI_lib_State_Machine.vi"("State(s) in (\"\")"=w312) -> ("States Out"=w311:string)  [unwired: 14 in]
      }
      frame "UI: Initialize" {
        # "#CSM \"UI: Initialize\"\nInitialize the User Interface, here.\n(this is called automatically, by the Macro: Init)"
        n132 = Unbundle By Name(w314) -> ("1.Ref.TabCtl"=w315:refnum<vi>[], "1.Ref.Pane"=w317:refnum<vi>)
        n133 = Bundle("TabCtl"=w315, "Pane"=w317, variant) -> (w316:T12)  [unwired: 1 in]
        n134 = call "Layout FGV.vi"("String"="Init", "InitRef"=w316) -> ()  [unwired: 10 in]
        n135 = call <vilib>:"Add State(s) to Queue__JKI_lib_State_Machine.vi"("State(s) in (\"\")"=w321) -> ("States Out"=w320:string)  [unwired: 14 in]
      }
      frame "UI: Save Layout" {
        n136 = call "Convert API String Arguments to Data.vim"("Reference Type"=path "", "API String"=w332) -> ("error out"=w325:errorcluster, "Data"=w324:path)  [unwired: 6 in]
        n137 = call <vilib>:"Clear Errors.vi"("error in (no error)"=w325) -> ()  [unwired: 5 in, 2 out]
        n138 = Empty String/Path?(string/path=w324) -> (empty?=w328:bool)
        n139 = Not(x=w328) -> (.not. x?=w327:bool)
        n140 = call <vilib>:"Check if File or Folder Exists.vi"("path"=w324) -> ("file or folder exists?"=w329:bool, "dup path"=w330:path)  [unwired: 8 in, 1 out]
        n141 = And(x=w329, y=w327) -> (x .and. y?=w326:bool)
        n142 = case shown="False" w326 {
          selector: w326 -> [_ w345]
          tunnel: [w341 w345] -> w322
          tunnel: [w343 w344] -> w323
          tunnel: w330 -> [_ w344]
          frame False {
            n143 = call "File Dialog2"("pattern (all files)"="*.Json", "pattern label"="Json") -> ("selected path"=w343:path, "cancelled"=w342:bool)  [unwired: 10 in, 2 out]
            n144 = Not(x=w342) -> (.not. x?=w341:bool)
          }
          frame True {
          }
        }
        n145 = case shown="False" w322 {
          tunnel: w323 -> [_ w337]
          frame False {
          }
          frame True {
            n146 = call "Layout FGV.vi"("String"="Save", "file (use dialog)"=w337) -> ()  [unwired: 10 in]
          }
        }
      }
      frame "UI: Load Layout" {
        n147 = call "Convert API String Arguments to Data.vim"("Reference Type"=path "", "API String"=w355) -> ("error out"=w351:errorcluster, "Data"=w349:path)  [unwired: 6 in]
        n148 = Empty String/Path?(string/path=w349) -> (empty?=w348:bool)
        n149 = call <vilib>:"Clear Errors.vi"("error in (no error)"=w351) -> ()  [unwired: 5 in, 2 out]
        n150 = Not(x=w348) -> (.not. x?=w347:bool)
        n151 = call <vilib>:"Check if File or Folder Exists.vi"("path"=w349) -> ("file or folder exists?"=w350:bool, "dup path"=w352:path)  [unwired: 8 in, 1 out]
        n152 = And(x=w350, y=w347) -> (x .and. y?=w346:bool)
        n153 = case shown="False" w346 {
          selector: w346 -> [_ w369]
          tunnel: [w367 w369] -> w354
          tunnel: [w366 w368] -> w353
          tunnel: w352 -> [_ w368]
          frame False {
            n154 = call "File Dialog"("pattern (all files)"="*.Json", "pattern label"="Json") -> ("selected path"=w366:path, "exists"=w367:bool, "error out"=w365:errorcluster)  [unwired: 10 in, 1 out]
            n155 = call <vilib>:"Clear Errors.vi"("error in (no error)"=w365) -> ()  [unwired: 5 in, 2 out]
          }
          frame True {
          }
        }
        n156 = case shown="True" w354 {
          tunnel: w353 -> [_ w361]
          frame False {
          }
          frame True {
            n157 = call "Layout FGV.vi"("String"="Load", "file (use dialog)"=w361) -> ()  [unwired: 10 in]
          }
        }
      }
      frame "UI: Cursor Set" {
        # "Argument"
        # "#CSM \"UI: Cursor Set\"\nSet and Unset Cursor Busy.\n(Usage: \"UI: Cursor Set >> Busy|Idle\")"
        n158 = disable-structure shown="Default" {
          disable-tunnel: [w377 _] -> w372
          disable-tunnel: w371 -> [w376 _]
          frame condition #0 (active) {
            n159 = case shown="\"Idle\", Default" w376 {
              tunnel: [w378 w379] -> w377
              frame "Idle", Default {
                n160 = call <vilib>:"Unset Busy.vi"() -> ("error out"=w378:errorcluster)  [unwired: 11 in]
              }
              frame "Busy" {
                n161 = call <vilib>:"Set Busy.vi"() -> ("error out"=w379:errorcluster)  [unwired: 10 in, 1 out]
              }
            }
          }
          frame condition #1 {
          }
        }
        n162 = call <vilib>:"Add State(s) to Queue__JKI_lib_State_Machine.vi"("State(s) in (\"\")"=w375) -> ("States Out"=w374:string)  [unwired: 14 in]
      }
      frame "UI: Front Panel State" {
        # "Argument"
        # "#CSM \"UI: Front Panel State\"\nSet Front Panel Open or Closed\n(Usage: \"UI: Front Panel State >> Open|Close\")"
        n163 = Unbundle By Name(w383) -> ("Core.Current VI Reference"=w382:refnum<vi>)
        n164 = case shown="\"Minimize\", \"Minimized\"" w381 {
          tunnel: [w393 w406 w417 w429 w441] -> w384
          tunnel: w382 -> [w392 w404 w416 w428 w440]
          frame "Open", "Standard", Default {
            w387 = T8."Standard" ("State")
            n165 = property class="VI"(reference=w392) -> (reference out=w390:refnum<vi>, error out=w391:errorcluster, "FP.State"=w389:T8)  [unwired: 1 in]
            n166 = Not Equal?(x=w389, y=w387) -> (x != y?=w388:bool)
            n167 = case shown="True" w388 {
              tunnel: [w397 w399] -> w393
              tunnel: w391 -> [w396 w399]
              tunnel: w390 -> [w395 _]
              tunnel: w387 -> [w394 _]
              frame True {
                n168 = invoke class="VI" method="FP.Open"(reference=w395, error in=w396, "Activate"=TRUE, "State"=w394) -> (error out=w397:errorcluster)  [unwired: 1 in, 4 out]
              }
              frame False {
              }
            }
          }
          frame "Close", "Closed" {
            n169 = property class="VI"(reference=w404) -> (reference out=w403:refnum<vi>, error out=w405:errorcluster, "FP.State"=w401:T8)  [unwired: 1 in]
            n170 = Not Equal?(x=w401, y=T8."Closed" ("Front Panel Window:State")) -> (x != y?=w400:bool)
            n171 = case shown="True" w400 {
              tunnel: [w407 w410] -> w406
              tunnel: w405 -> [w407 w409]
              tunnel: w403 -> [_ w408]
              frame False {
              }
              frame True {
                n172 = invoke class="VI" method="FP.Close"(reference=w408, error in=w409) -> (error out=w410:errorcluster)  [unwired: 1 in, 2 out]
              }
            }
          }
          frame "Hidden", "Hide" {
            w411 = T8."Hidden" ("State")
            n173 = property class="VI"(reference=w416) -> (reference out=w414:refnum<vi>, error out=w415:errorcluster, "FP.State"=w413:T8)  [unwired: 1 in]
            n174 = Not Equal?(x=w413, y=w411) -> (x != y?=w412:bool)
            n175 = case shown="True" w412 {
              tunnel: [w421 w422] -> w417
              tunnel: w415 -> [w420 w422]
              tunnel: w414 -> [w419 _]
              tunnel: w411 -> [w418 _]
              frame True {
                n176 = invoke class="VI" method="FP.Open"(reference=w419, error in=w420, "State"=w418) -> (error out=w421:errorcluster)  [unwired: 2 in, 4 out]
              }
              frame False {
              }
            }
          }
          frame "Minimize", "Minimized" {
            w423 = T8."Minimized" ("State")
            n177 = property class="VI"(reference=w428) -> (reference out=w426:refnum<vi>, error out=w427:errorcluster, "FP.State"=w425:T8)  [unwired: 1 in]
            n178 = Not Equal?(x=w425, y=w423) -> (x != y?=w424:bool)
            n179 = case shown="False" w424 {
              tunnel: [w433 w434] -> w429
              tunnel: w427 -> [w432 w434]
              tunnel: w426 -> [w431 _]
              tunnel: w423 -> [w430 _]
              frame True {
                n180 = invoke class="VI" method="FP.Open"(reference=w431, error in=w432, "State"=w430) -> (error out=w433:errorcluster)  [unwired: 2 in, 4 out]
              }
              frame False {
              }
            }
          }
          frame "Maximize", "Maximized" {
            w435 = T8."Maximized" ("State")
            n181 = property class="VI"(reference=w440) -> (reference out=w438:refnum<vi>, error out=w439:errorcluster, "FP.State"=w437:T8)  [unwired: 1 in]
            n182 = Not Equal?(x=w437, y=w435) -> (x != y?=w436:bool)
            n183 = case shown="True" w436 {
              tunnel: [w445 w446] -> w441
              tunnel: w439 -> [w444 w446]
              tunnel: w438 -> [w443 _]
              tunnel: w435 -> [w442 _]
              frame True {
                n184 = invoke class="VI" method="FP.Open"(reference=w443, error in=w444, "State"=w442) -> (error out=w445:errorcluster)  [unwired: 2 in, 4 out]
              }
              frame False {
              }
            }
          }
        }
        n185 = call <vilib>:"Add State(s) to Queue__JKI_lib_State_Machine.vi"("State(s) in (\"\")"=w386) -> ("States Out"=w385:string)  [unwired: 14 in]
      }
      frame "---------- Macro ----------" {
        # "#CSM \"Category Seperator\"\nDo not put any code in this frame."
        n186 = call <vilib>:"Add State(s) to Queue__JKI_lib_State_Machine.vi"("State(s) in (\"\")"=w450) -> ("States Out"=w449:string)  [unwired: 14 in]
      }
      frame "Macro: Initialize" {
        w452 = "Data: Initialize\nInitialize Core Data\nUI: Initialize\nUI: Front Panel State >> Maximize\nEvents: Register\n//UI: Front Panel State >> Open"  # Data: Initialize Initialize Core Data UI: Initialize UI: Front Panel State >> Maximize Events: Register //UI: Front Panel State >> Open
        # "#CSM \"Macro: Initialize\"\nInitialization Macro (This is called once, when the VI starts)"
        n187 = call <vilib>:"Add State(s) to Queue__JKI_lib_State_Machine.vi"("State(s) in Front (\"\")"=w452, "State(s) in (\"\")"=w455) -> ("States Out"=w454:string)  [unwired: 13 in]
      }
      frame "Macro: Exit" {
        # "#CSM \"Macro: Exit\"\nExit Macro (This is called once, when the VI exits)"
        n188 = Unbundle By Name(w464) -> ("Core.Close Panel on Exit?"=w463:bool)
        n189 = Select(t="UI: Front Panel State >> Close", s=w463, f="") -> (s? t:f=w460:string)
        n190 = call <vilib>:"Add State(s) to Queue__JKI_lib_State_Machine.vi"("State(s) in Front (\"\")"="//Exit Sub-Modules ", "State(s) in (\"\")"=w460, "State(s) at Back (\"\")"="Data: Cleanup\nEvents: Unregister\nExit") -> ("States Out"=w458:string)  [unwired: 12 in]
        n191 = call <vilib>:"Add State(s) to Queue__JKI_lib_State_Machine.vi"("State(s) in Front (\"\")"=w458, "State(s) in (\"\")"=w466) -> ("States Out"=w465:string)  [unwired: 13 in]
      }
      frame "---------- API ----------" {
        # "#CSM \"Category Seperator\"\nDo not put any code in this frame."
      }
      frame "API: UpdateViewList" {
        # "#CSM API Example\nCopy/Rename this case for your own API"
        n192 = call "Convert API String Arguments to Data.vim"("Reference Type"=T4[] [], "API String"=w475) -> ("Data"=w470:T4[])  [unwired: 6 in, 1 out]
        n193 = call "Layout FGV.vi"("String"="Set", "Variant"=w470, "name"="ViewList") -> ()  [unwired: 9 in]
        n194 = Bundle By Name(cluster=w477, "1.Val.UpdateInsertableVI"=w470) -> (w473:T7)
      }
      frame "API: Hello" {
        # "#CSM API Example\nCopy/Rename this case for your own API"
        n195 = Empty String/Path?(string/path=w480) -> (empty?=w479:bool)
        n196 = case shown="False" w479 {
          tunnel: w480 -> [w484 _]
          frame False {
            n197 = One Button Dialog(message=w484) -> ()  [unwired: 1 in, 1 out]
          }
          frame True {
          }
        }
      }
      frame "API: SubpanelUpdate" {
        # "#CSM API Example\nCopy/Rename this case for your own API"
        n198 = control-ref of="Sub Panel"() -> (w492:refnum<vi>)
        n199 = Unbundle By Name(w489) -> ("Core.Current VI Reference"=w488:refnum<vi>)
        n200 = call "Convert API String Arguments to Data.vim"("Reference Type"=w492, "API String"=w493) -> ("Data"=w486:refnum<vi>)  [unwired: 6 in, 1 out]
        n201 = property class="SubPnl"(reference=w486) -> ("OwningVI"=w485:refnum<vi>)  [unwired: 1 in, 2 out]
        n202 = invoke on="Invoke Node" class="VI" method="FP.Close"(reference=w488) -> (reference out=w490:refnum<vi>, error out=w491:errorcluster)  [unwired: 2 in, 1 out]
        n203 = invoke on="Invoke Node" class="SubPnl" method="Insert VI"(reference=w486, error in=w491, "VI Ref"=w490) -> ()  [unwired: 1 in, 4 out]
        n204 = Bundle By Name(cluster=w489, "1.Ref.Owning VI"=w485) -> (w487:T7)
      }
      frame "---------- Action ----------" {
        # "#CSM \"Category Seperator\"\nDo not put any code in this frame."
        n205 = call <vilib>:"Add State(s) to Queue__JKI_lib_State_Machine.vi"("State(s) in (\"\")"=w499) -> ("States Out"=w498:string)  [unwired: 14 in]
      }
      frame "Action: action1" {
        # "#CSM \"Internal State\"\nThis category is used for holding internal states"
        n206 = call <vilib>:"Add State(s) to Queue__JKI_lib_State_Machine.vi"("State(s) in (\"\")"=w503) -> ("States Out"=w502:string)  [unwired: 14 in]
      }
      frame "Action: action2" {
        # "#CSM \"Internal State\"\nThis category is used for holding internal states"
        n207 = call <vilib>:"Add State(s) to Queue__JKI_lib_State_Machine.vi"("State(s) in (\"\")"=w507) -> ("States Out"=w506:string)  [unwired: 14 in]
      }
    }
  }
